vi "Sample_Dialog.vi"(8 "Script":path, 9 "Type":string, 10 "Name":string, 11 "ID":string) -> (1 "Canceled?":bool, 2 "AnalysisData Out":string[](array[string]))   [LabVIEW 2013]
doc: "Dialo that asks for the SampleInformation\nID\nName\nType\nScript Path\n\nThose values can be prescribed if necessary"
panel:
  out "error out":errorcluster
  in  "error in (no error)":errorcluster
  in  "Cancel Button":bool
  in  "Okay button":bool
  # "Analysis Information"
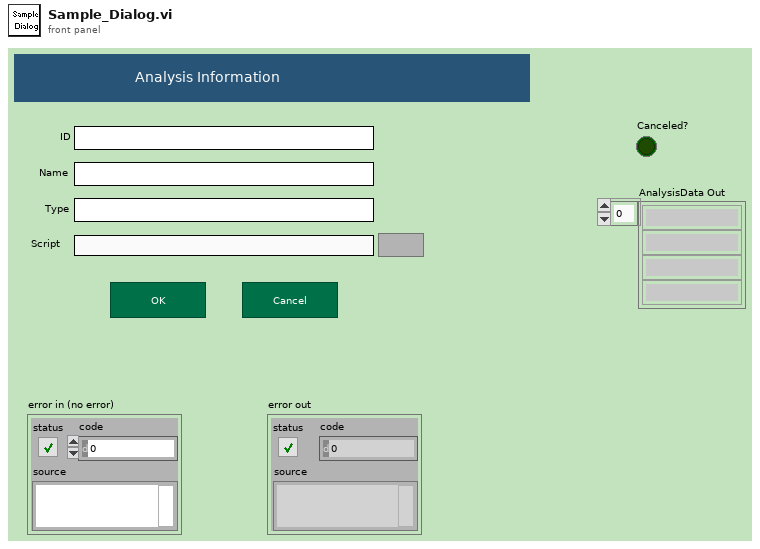
[diagram p1: front panel]
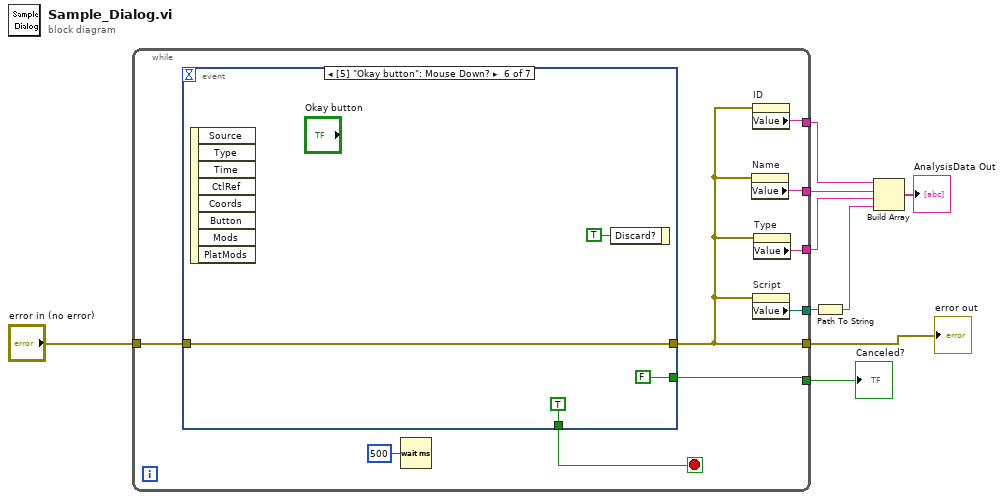
[diagram p0: block diagram]
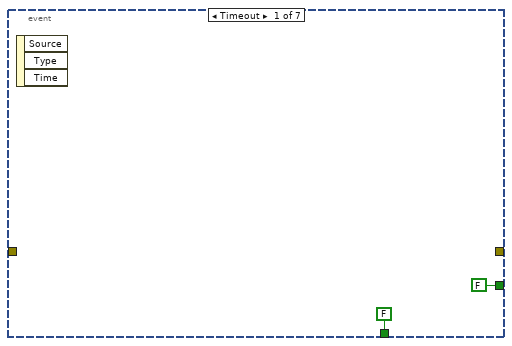
[diagram p2: hidden frame]
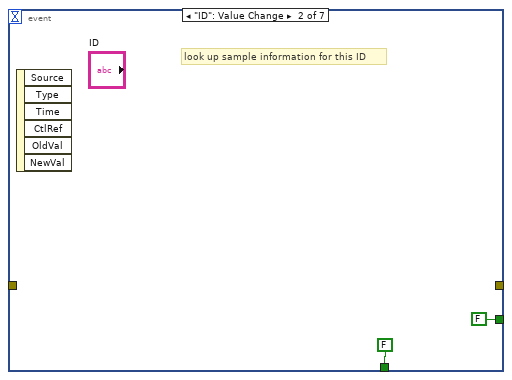
[diagram p3: hidden frame]
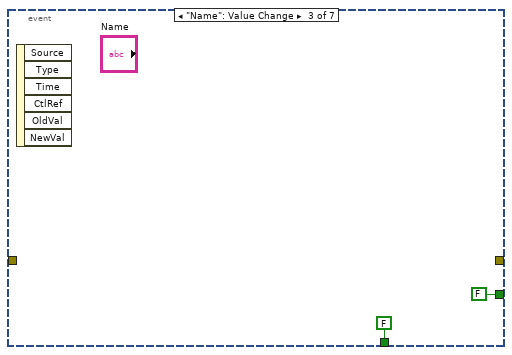
[diagram p4: hidden frame]
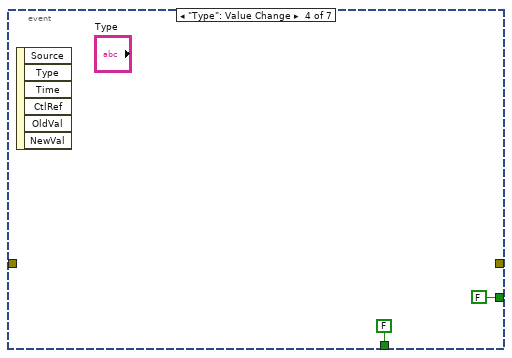
[diagram p5: hidden frame]
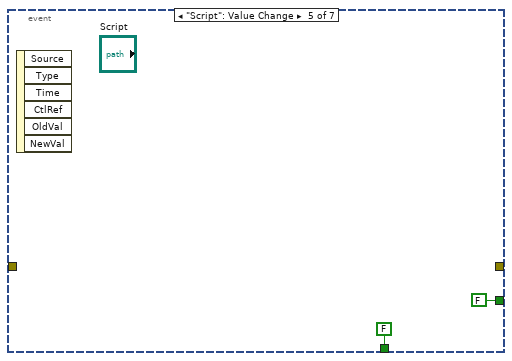
[diagram p6: hidden frame]
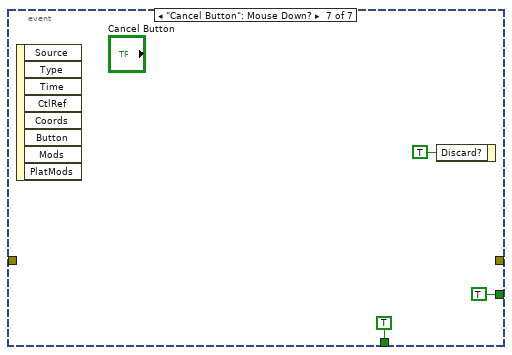
[diagram p7: hidden frame]
diagram:
  n1 = while {
    tunnel: [w14] -> w8
    tunnel: [w13] -> w7
    tunnel: [w12] -> w6
    tunnel: [w15] -> w9
    tunnel: [w16] -> w3
    tunnel: "error in (no error)" -> [w11]
    tunnel: [w10] -> w1
    stop <- w18 stop-if-true
    n2 = event shown="[5] \"Okay button\": Mouse Down?" {
      selector: _ -> [_ _ _ _ _ _ _]
      dyn-events: _ -> [_ _ _ _ _ _ _]
      timeout: _ -> [_ _ _ _ _ _ _]
      tunnel: [FALSE FALSE FALSE FALSE FALSE TRUE TRUE] -> w18
      tunnel: [FALSE FALSE FALSE FALSE FALSE FALSE TRUE] -> w16
      tunnel: w11 -> [_ _ _ _ _ w29 _]
      tunnel: [_ _ _ _ _ w29 _] -> w10
      event Timeout {
        n3 = event-data() -> ()  [unwired: 1 in, 3 out]
      }
      event "ID": Value Change {
        # "look up sample information for this ID"
        n4 = event-data() -> ()  [unwired: 1 in, 6 out]
      }
      event "Name": Value Change {
        n5 = event-data() -> ()  [unwired: 1 in, 6 out]
      }
      event "Type": Value Change {
        n6 = event-data() -> ()  [unwired: 1 in, 6 out]
      }
      event "Script": Value Change {
        n7 = event-data() -> ()  [unwired: 1 in, 6 out]
      }
      event "Okay button": Mouse Down? {
        n8 = event-data() -> ()  [unwired: 1 in, 8 out]
        n9 = event-data("Discard?"=TRUE) -> ()  [unwired: 1 in, 1 out]
      }
      event "Cancel Button": Mouse Down? {
        n10 = event-data() -> ()  [unwired: 1 in, 8 out]
        n11 = event-data("Discard?"=TRUE) -> ()  [unwired: 1 in, 1 out]
      }
    }
    n12 = Wait (ms)(milliseconds to wait=u32 500) -> ()  [unwired: 1 out]
    n13 = property on="Name" class="Str"(error in=w10) -> ("Value"=w14:string)  [unwired: 1 in, 2 out]
    n14 = property on="ID" class="Str"(error in=w10) -> ("Value"=w15:string)  [unwired: 1 in, 2 out]
    n15 = property on="Script" class="Path"(error in=w10) -> ("Value"=w12:path)  [unwired: 1 in, 2 out]
    n16 = property on="Type" class="Str"(error in=w10) -> ("Value"=w13:string)  [unwired: 1 in, 2 out]
  }
  "Canceled?" <- w3
  "error out" <- w1
  n17 = Path To String(path=w6) -> (string=w5:string)
  n18 = Build Array(w9, w8, w7, w5) -> (→"AnalysisData Out":string[])
